vi "WPI_IMU_Loop.vi"(8 "error in":errorcluster, 11 "ADI IMU Interrupt DevRef":T1={"SimpleGyroDevRef"={"DevStatus"={"status"=FALSE, "code"=0, "source"=""}, "Handle"=0, "SPI Bus"=enum."SPI On-Board, CS0", "Device Found"=FALSE, "Sample Rate"=0.0, "Device Ready"=FALSE, "Yaw Axis"=enum."Z", "AHRS Algorithm"=enum."Complementary"}, "InterruptRef"={"DevStatus"={"status"=FALSE, "code"=0, "source"=""}, "InterruptIndex"=enum."0"}} {"SimpleGyroDevRef"."Sample Rate" min=0.25 max=100.0 step=0.25}) -> (0 "error out":errorcluster)   [LabVIEW 2015, in "FRC ADI MXP IMU.lvlib"]
doc: "Periodically reads the ADI MXP IMU valuse and makes data available for use elsewhere in your robot project. Place this block within PeriodicTasks.vi outside any loops."
uses:
  FRC ADI MXP IMU.lvlib
  WPI_AnalogDevicesIMUInterruptDevRef.ctl
  WPI_AnalogDevicesIMUDevRef.ctl
  <vilib>/Rock Robotics/SystemInterfaces/spilib/spi_bus.ctl
  <vilib>/Rock Robotics/WPI/Interrupt/WPI_InterruptRef.ctl
  <vilib>/Rock Robotics/SystemInterfaces/Interrupt/FPGA_InterruptIndex.ctl
  <vilib>/Rock Robotics/WPI/SPI/WPI_SPIDevRef.ctl
  <vilib>/Platform/TimedLoop/XDataNode/timing_clust.ctl
  <vilib>/Platform/TimedLoop/XDataNode/nitl_modes.ctl
  <vilib>/Platform/TimedLoop/XDataNode/wakeup.ctl
  <vilib>/Rock Robotics/SystemInterfaces/Interrupt/FPGA_WaitOnInterrupt.vi
  <vilib>/Rock Robotics/WPI/Utilities/WPI_UtilitiesTimebaseConstants.vi
  <vilib>/Rock Robotics/SystemInterfaces/Interrupt/FPGA_InterruptReadTimestamp.vi
  <vilib>/platform/TimedLoop/XDataNode/XDataNode.xnode
  <vilib>/ptbypt/NI_PtbyPt.lvlib
  <vilib>/Platform/TimedLoop/XDataNode/XDNodeRunTimeDep.lvlib
panel:
  out "Device Found":bool
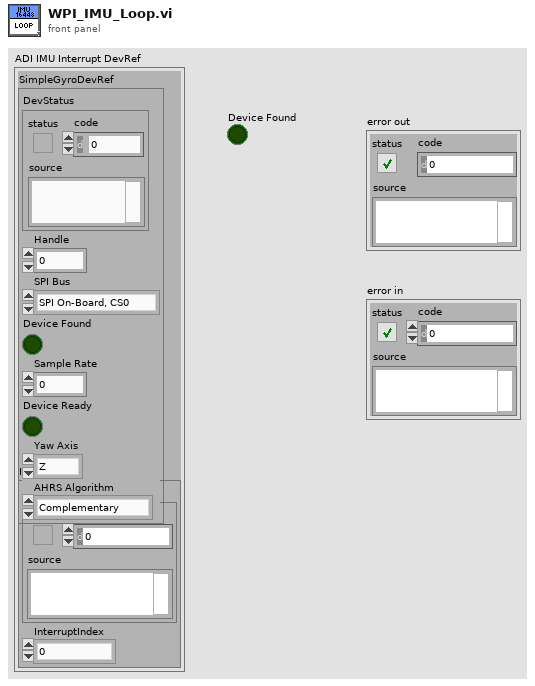
[diagram p1: front panel]
types:
  T1 = typedef "FRC ADI MXP IMU.lvlib/WPI_AnalogDevicesIMUInterruptDevRef.ctl" = cluster{"SimpleGyroDevRef":T2, "InterruptRef":T4}
  T2 = typedef "FRC ADI MXP IMU.lvlib/WPI_AnalogDevicesIMUDevRef.ctl" = cluster{"DevStatus":errorcluster, "Handle":i32, "SPI Bus":T3, "Device Found":bool, "Sample Rate":dbl, "Device Ready":bool, "Yaw Axis":enum16{"X", "Y", "Z"}, "AHRS Algorithm":enum16{"Complementary", "Madgwick"}}
  T3 = typedef "spi_bus.ctl" = enum16{"SPI On-Board, CS0", "SPI On-Board, CS1", "SPI On-Board, CS2", "SPI On-Board, CS3", "SPI MXP", "Invalid"}
  T4 = typedef "WPI_InterruptRef.ctl" = cluster{"DevStatus":errorcluster, "InterruptIndex":T5}
  T5 = typedef "FPGA_InterruptIndex.ctl" = enum8{"0", "1", "2", "3", "4", "5", "6", "7", "Invalid"}
  T6 = typedef "WPI_SPIDevRef.ctl" = cluster{"DevStatus":errorcluster, "Handle":i32, "SPI Bus":T3}
  T7 = cluster{"Output[0]":dbl, "Output[1]":dbl, "Output[2]":dbl}
  T8 = typedef "XDNodeRunTimeDep.lvlib/timing_clust.ctl" = cluster{"Expected End [f-1]":u64, "Actual End [f-1]":u64, "Finished Late? [f-1]":bool, "Expected End [i-1]":u64, "Actual End [i-1]":u64, "Finished Late? [i-1]":bool, "Expected Start [i]":u64, "Actual Start [i]":u64, "Expected Start [f]":u64, "Actual Start [f]":u64, "Source Name":string, "Structure Name":string, "Period":i64, "Deadline":i64, "Offset":i64, "Start":i64, "Priority":i32, "Timeout":i32, "Mode":T9, "Wakeup Reason":T10, "Error":errorcluster, "Source Type":string, "Secondary Source Type":string, "Global End Time":u64, "Global Start Time":u64, "Frame Duration":u64, "Iteration Duration":u64, "Assigned CPU":i32, "I/O Scan Engine Mode":u32}
  T9 = typedef "XDNodeRunTimeDep.lvlib/nitl_modes.ctl" = enum32{"No Change", "Process missed periods, maintain original phase", "Discard missed periods, maintain original phase", "Process missed periods, ignore original phase", "Discard missed periods, ignore original phase"}
  T10 = typedef "XDNodeRunTimeDep.lvlib/wakeup.ctl" = enum32{"Normal", "Aborted", "Asynchronous wakeup", "Timing source error", "Timed loop error", "Timeout"}
  T11 = cluster{"Data Array[0]":dbl, "Data Array[1]":dbl, "Data Array[2]":dbl, "Data Array[3]":dbl, "Data Array[4]":dbl, "Data Array[5]":dbl, "Data Array[6]":dbl, "Data Array[7]":dbl, "Data Array[8]":dbl, "Data Array[9]":dbl, "Data Array[10]":dbl}
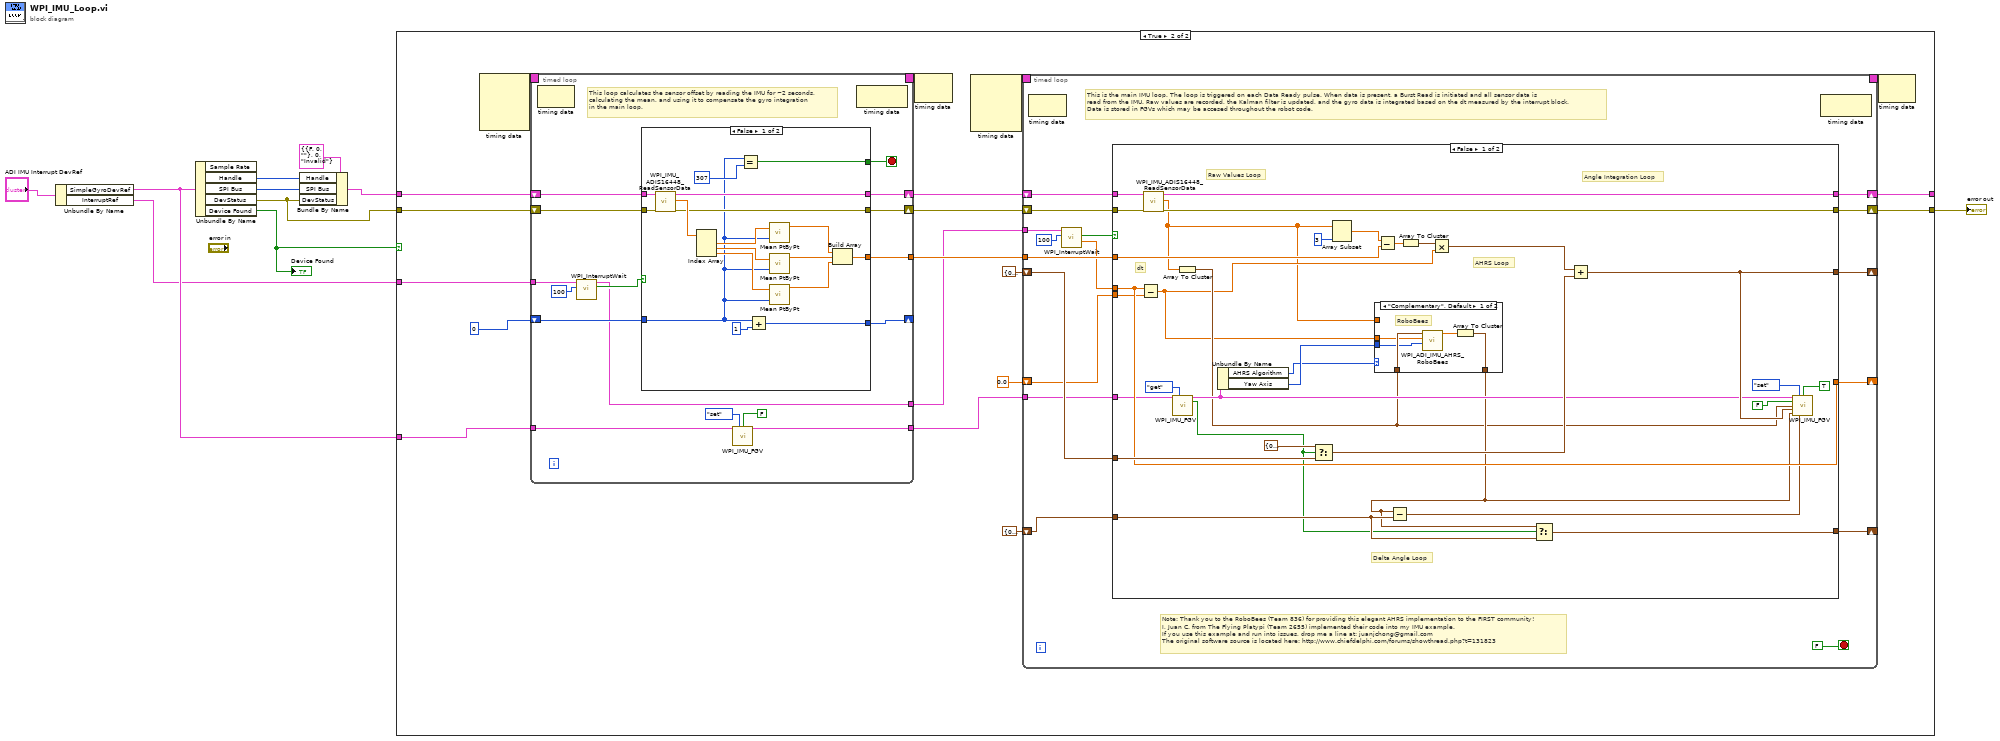
[diagram p0: block diagram]
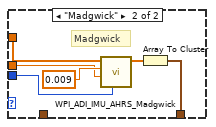
[diagram p3: hidden frame]
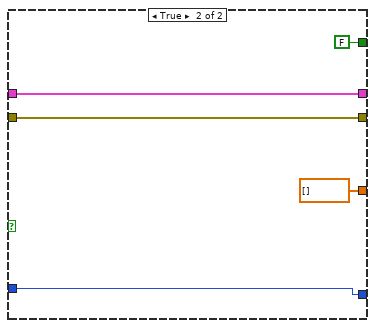
[diagram p5: hidden frame]
diagram:
  n1 = Unbundle By Name("ADI IMU Interrupt DevRef") -> ("SimpleGyroDevRef"=w2:T2, "InterruptRef"=w1:T4)
  n2 = Unbundle By Name(w2) -> ("Handle"=w9:i32, "SPI Bus"=w8:T3, "DevStatus"=w5:errorcluster, "Device Found"=w7:bool)  [unwired: 1 out]
  "Device Found" <- w7
  n3 = Bundle By Name(cluster=T6 {"DevStatus"={"status"=FALSE, "code"=0, "source"=""}, "Handle"=0, "SPI Bus"=enum."Invalid"} ("SPIDevRef out"), "Handle"=w9, "SPI Bus"=w8, "DevStatus"=w5) -> (w6:T6)
  n4 = case shown="True" w7 {
    tunnel: w6 -> [w12 w29]
    tunnel: w5 -> [w11 w28]
    tunnel: [w11 w31] -> w4
    tunnel: [w12 w30] -> _
    tunnel: w2 -> [_ w16]
    tunnel: w1 -> [_ w18]
    frame False {
    }
    frame True {
      n5 = node-c288() -> (w20:T8)  [unwired: 4 in]
      n6 = timed-loop {
        tunnel: [w113] -> w24
        shift-right: [w115] -> w26
        shift-left: w29 -> [w107]
        shift-right: [w116] -> w27
        shift-left: w28 -> [w106]
        shift-right: [w111] -> _
        shift-left: 0 -> [w112]
        tunnel: w18 -> [w110]
        tunnel: [w105] -> w22
        timing: w20 -> [_]
        timing-out: [_] -> w19
        tunnel: w16 -> [w103]
        tunnel: [w104] -> w13
        stop <- w114 stop-if-true
        # "This loop calculates the sensor offset by reading the IMU for ~2 seconds, \ncalculating the mean, and using it to compensate the gyro integration\nin the main loop."
        n7 = node-c288() -> ()  [unwired: 1 in, 1 out]
        n8 = call <vilib>:"WPI_InterruptWait.vi"("Timeout (ms)"=100, "InterruptRef"=w110) -> ("Timed Out"=w108:bool, "InterruptRef"=w105:T4)  [unwired: 5 in, 3 out]
        n9 = case shown="False" w108 {
          tunnel: [w134 w137] -> w116
          tunnel: [w133 w138] -> w115
          tunnel: [w128 FALSE] -> w114
          tunnel: [w124 dbl[] []] -> w113
          tunnel: w106 -> [w123 w137]
          tunnel: w107 -> [w122 w138]
          tunnel: w112 -> [w119 w140]
          tunnel: [w121 w140] -> w111
          frame False {
            n10 = call "WPI_IMU_ADIS16448_ReadSensorData.vi"("error in (no error)"=w123, "SPIDevRef in"=w122) -> ("error out"=w134:errorcluster, "Data Array"=w135:dbl[], "SPIDevRef out"=w133:T6)  [unwired: 7 in]
            n11 = Index Array(array=w135) -> (element #1=w132:dbl, element #2=w131:dbl, element #3=w130:dbl)  [unwired: 3 in]
            n12 = Equal?(x=w119, y=307) -> (x = y?=w128:bool)
            n13 = Add(x=w119, y=1) -> (x+y=w121:i32)
            n14 = call <vilib>:"Mean PtByPt.vi"("x"=w132, "sample length"=w119) -> ("mean"=w127:dbl)  [unwired: 2 in, 1 out]
            n15 = call <vilib>:"Mean PtByPt.vi"("x"=w131, "sample length"=w119) -> ("mean"=w126:dbl)  [unwired: 2 in, 1 out]
            n16 = call <vilib>:"Mean PtByPt.vi"("x"=w130, "sample length"=w119) -> ("mean"=w125:dbl)  [unwired: 2 in, 1 out]
            n17 = Build Array(w127, w126, w125) -> (w124:dbl[])
          }
          frame True {
          }
        }
        n18 = call "WPI_IMU_FGV.vi"("SimpleGyroDevRef"=w103, "Operation"=enum16{"set", "get"}."set", "Sensor Ready?"=FALSE) -> ("SimpleGyroDevRef"=w104:T2)  [unwired: 6 in, 6 out]
        n19 = node-c288() -> ()  [unwired: 1 in, 1 out]
      }
      n20 = node-c288(w19) -> ()  [unwired: 1 out]
      n21 = node-c288() -> (w15:T8)  [unwired: 4 in]
      n22 = timed-loop {
        shift-right: [w48] -> w30
        shift-left: w26 -> [w42]
        shift-right: [w47] -> w31
        shift-left: w27 -> [w41]
        shift-right: [w45] -> _
        shift-left: cluster{dbl, dbl, dbl} {0.0, 0.0, 0.0} -> [w44]
        tunnel: w24 -> [w43]
        tunnel: w22 -> [w39]
        shift-right: [w37] -> _
        shift-left: 0.0 ("TimeStamp") -> [w36]
        shift-right: [w33] -> _
        shift-left: T7 {"Output[0]"=0.0, "Output[1]"=0.0, "Output[2]"=0.0} -> [w35]
        tunnel: w13 -> [w32]
        timing: w15 -> [_]
        timing-out: [_] -> w14
        stop <- FALSE stop-if-true
        # "Note: Thank you to the RoboBees (Team 836) for providing this elegant AHRS implementation to the FIRST community!\nI, Juan C. from The Flying Platypi (Team 2655) implemented their code into my IMU example.\nIf you use this example and run into issues, drop me a line at: juanjchong@gmail.com\nThe original software source is located here: http://www.chiefdelphi.com/forums/showthread.php?t=131823"
        # "This is the main IMU loop. The loop is triggered on each Data Ready pulse. When data is present, a Burst Read is initiated and all sensor data is \nread from the IMU. Raw values are recorded, the Kalman filter is updated, and the gyro data is integrated based on the dt measured by the interrupt block.\nData is stored in FGVs which may be accesed throughout the robot code."
        n23 = node-c288() -> ()  [unwired: 1 in, 1 out]
        n24 = call <vilib>:"WPI_InterruptWait.vi"("Timeout (ms)"=100, "InterruptRef"=w39) -> ("TimeStamp"=w38:dbl, "Timed Out"=w34:bool)  [unwired: 5 in, 3 out]
        n25 = case shown="False" w34 {
          tunnel: w42 -> [w82 w98]
          tunnel: w41 -> [w81 w97]
          tunnel: [w80 w98] -> w48
          tunnel: [w79 w97] -> w47
          tunnel: w32 -> [w60 _]
          tunnel: [w72 w96] -> w45
          tunnel: w44 -> [w75 w96]
          tunnel: w43 -> [w70 _]
          tunnel: w38 -> [w66 _]
          tunnel: [w66 w95] -> w37
          tunnel: w36 -> [w65 w95]
          tunnel: w35 -> [w63 w94]
          tunnel: [w62 w94] -> w33
          frame False {
            # "Delta Angle Loop"
            # "dt"
            # "Angle Integration Loop"
            # "AHRS Loop"
            # "Raw Values Loop"
            n26 = Subtract(x=w66, y=w65) -> (x-y=w54:dbl)
            n27 = call "WPI_IMU_ADIS16448_ReadSensorData.vi"("error in (no error)"=w81, "SPIDevRef in"=w82) -> ("error out"=w79:errorcluster, "Data Array"=w52:dbl[], "SPIDevRef out"=w80:T6)  [unwired: 7 in]
            n28 = call "WPI_IMU_FGV.vi"("SimpleGyroDevRef"=w60, "Operation"=enum16{"set", "get"}."get") -> ("SimpleGyroDevRef"=w57:T2, "Reset Out"=w59:bool)  [unwired: 7 in, 5 out]
            n29 = Array To Cluster(array=w52) -> (cluster=w55:T11)
            n30 = Unbundle By Name(w57) -> ("AHRS Algorithm"=w51:enum16{"Complementary", "Madgwick"}, "Yaw Axis"=w53:enum16{"X", "Y", "Z"})
            n31 = Select(t=T7 {"Output[0]"=0.0, "Output[1]"=0.0, "Output[2]"=0.0} ("cluster"), s=w59, f=w75) -> (s? t:f=w74:T7)
            n32 = Array Subset(array=w52, length=3) -> (w71:dbl[])  [unwired: 1 in]
            n33 = case shown="\"Complementary\", Default" w51 {
              tunnel: [w86 w91] -> w56
              tunnel: w55 -> [w85 _]
              tunnel: w54 -> [w84 w90]
              tunnel: w53 -> [w83 w88]
              tunnel: w52 -> [_ w89]
              frame "Complementary", Default {
                # "RoboBees"
                n34 = call "WPI_ADI_IMU_AHRS_RoboBees.vi"("Yaw Axis"=w83, "dt (s)"=w84, "IMU Rates"=w85) -> ("Output"=w87:dbl[])  [unwired: 4 in, 3 out]
                n35 = Array To Cluster(array=w87) -> (cluster=w86:T7)
              }
              frame "Madgwick" {
                # "Madgwick"
                n36 = call "WPI_ADI_IMU_AHRS_Madgwick.vi"("Yaw Axis"=w88, "dt (s)"=w90, "Beta"=0.009, "Data"=w89) -> ("Output"=w92:dbl[])  [unwired: 7 in]
                n37 = Array To Cluster(array=w92) -> (cluster=w91:T7)
              }
            }
            n38 = Subtract(x=w71, y=w70) -> (x-y=w69:dbl[])
            n39 = Subtract(x=w56, y=w63) -> (x-y=w64:T7)
            n40 = Array To Cluster(array=w69) -> (cluster=w68:cluster{"[0]":dbl, "[1]":dbl, "[2]":dbl})
            n41 = Multiply(x=w68, y=w54) -> (x*y=w67:cluster{"[0]":dbl, "[1]":dbl, "[2]":dbl})
            n42 = Select(t=w56, s=w59, f=w63) -> (s? t:f=w62:T7)
            n43 = Add(x=w67, y=w74) -> (x+y=w72:cluster{dbl, dbl, dbl})
            n44 = call "WPI_IMU_FGV.vi"("SimpleGyroDevRef"=w57, "Operation"=enum16{"set", "get"}."set", "Sensor Ready?"=TRUE, "Reset"=FALSE ("Calibrated"), "IMU Data"=w55, "IMU Angles"=w72, "IMU AHRS"=w56, "IMU AHRS DELTA"=w64) -> ()  [unwired: 1 in, 7 out]
          }
          frame True {
            # "Waiting for an interrupt..."
          }
        }
        n45 = node-c288() -> ()  [unwired: 1 in, 1 out]
      }
      n46 = node-c288(w14) -> ()  [unwired: 1 out]
    }
  }
  "error out" <- w4
